vi "zx shift for round-trip-2 (SubVI).vi"(11 "input":u16[][][](array[numeric])) -> (3 "output":u16[][][](array[numeric]))   [LabVIEW 2024]
uses:
  Global variables/global for picoscope.vi
  <vilib>/gmath/interp.llb/Interpolate 2D (1d xi,yi).vi
  <vilib>/gmath/NI_Gmath.lvlib
panel:
  in  "use local settings":bool
  in  "z shift":dbl format="%_3g"
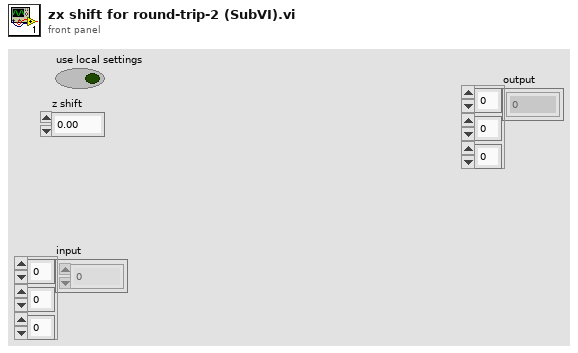
[diagram p1: front panel]
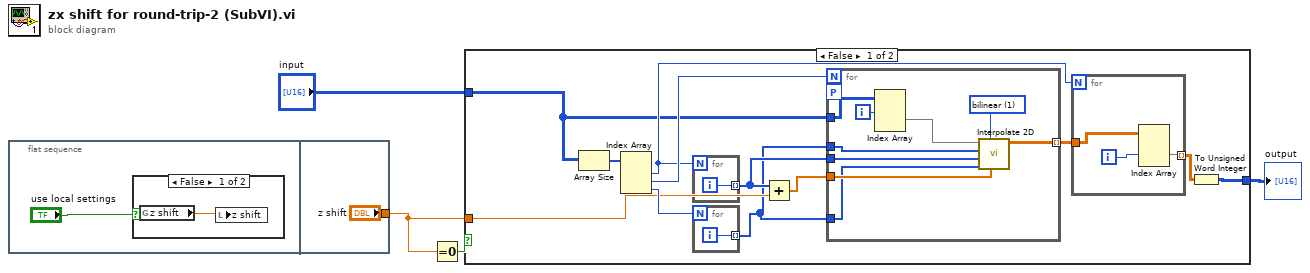
[diagram p0: block diagram]
diagram:
  n1 = flat-sequence {
    tunnel: ["z shift"] -> w2
    frame #0 {
      n2 = case shown="False" "use local settings" {
        frame False {
          n3 = global read "global for picoscope.vi" "z shift"() -> (w6:dbl)
          n4 = local write "z shift"(w6) -> ()
        }
        frame True {
        }
      }
    }
    frame #1 {
    }
  }
  n5 = Equal To 0?(x=w2) -> (x = 0?=w1:bool)
  n6 = case shown="False" w1 {
    tunnel: "input" -> [w9 w34]
    tunnel: [w10 w34] -> w3
    tunnel: w2 -> [w11 _]
    frame False {
      n7 = Array Size(array=w9) -> (size(s)=w19:i32[])
      n8 = Index Array(array=w19) -> (element #1=w14:i32, element #2=w18:i32, element #3=w13:i32)  [unwired: 3 in]
      n9 = for {
        N: w14 -> [_]
        tunnel: [w24] -> w17 mode=indexing
        i -> [w24]
      }
      n10 = for {
        N: w13 -> [_]
        tunnel: [w23] -> w8 mode=indexing
        i -> [w23]
      }
      n11 = Add(x=w17, y=w11) -> (x+y=w16:dbl[])
      n12 = for {
        N: w18 -> [_]
        tunnel: w17 -> [w33]
        tunnel: w8 -> [w32]
        tunnel: w16 -> [w31]
        tunnel: w8 -> [w30]
        tunnel: w9 -> [w29]
        tunnel: [w26] -> w15 mode=indexing
        workers-P: _ -> [_]
        i -> [w28]
        w25 = 1 items=["nearest", "bilinear", "bicubic", "bicubic spline"] ("method")
        n13 = Index Array(array=w29, index (dim 1)=w28) -> (element=w27:u16[][])  [unwired: 2 in]
        n14 = call-poly <vilib>:"Interpolate 2D.vi"("yi"=w31, "method"=w25, "xi"=w30, "Y"=w33, "X"=w32, "Z"=w27) -> ("zi"=w26:dbl[][])  [unwired: 2 in, 3 out]
      }
      n15 = for {
        N: w14 -> [_]
        tunnel: w15 -> [w22]
        tunnel: [w20] -> w12 mode=indexing
        i -> [w21]
        n16 = Index Array(array=w22, index (dim 1)=w21) -> (element=w20:dbl[][])  [unwired: 2 in]
      }
      n17 = To Unsigned Word Integer(number=w12) -> (unsigned 16bit integer=w10:u16[][][])
    }
    frame True {
    }
  }
  "output" <- w3
